vi "agilent_reader.vi"(0 "Action":u8(ring)=1 items=["read new values"=1, "read last values "=2], 5 "Voltage Readings":u16=3, 7 "Temperature Readings":u16=1) -> (1 "Burette Temp Average":dbl, 2 "Cell Temp":dbl, 3 "Acid Temp":dbl, 4 "Burette Temp 1":dbl, 6 "Burette Temp 2":dbl, 8 "Room Temp":dbl, 10 "Voltage 1":dbl, 11 "Data Cluster":T1, 12 "Voltage 1 StandDev":dbl, 13 "Voltage 2 StandDev":dbl, 14 "Average Voltage":dbl, 15 "Voltage 2":dbl)   [LabVIEW 2010]
doc: "This VI is a wrapper for the agilent_action_engine vi's \"read\" action. It makes spitting out the values you need just a bit easier. Just pass in the number of readings for both voltage and temp and do what you will with the resulting data."
uses:
  ProbeClass/TempProbeSet.lvclass
  <vilib>/Analysis/NI_AALBase.lvlib
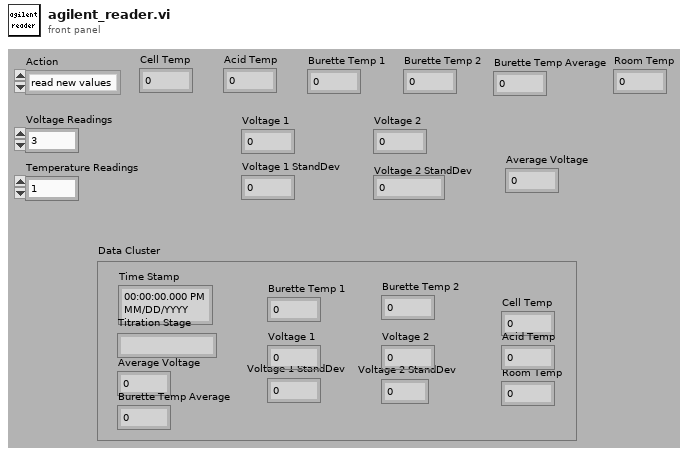
[diagram p1: front panel]
types:
  T1 = cluster{"Time Stamp":timestamp, "Titration Stage":string, "Average Voltage":dbl, "Burette Temp Average":dbl, "Voltage 1":dbl, "Voltage 2":dbl, "Voltage 1 StandDev":dbl, "Voltage 2 StandDev":dbl, "Burette Temp 1":dbl, "Burette Temp 2":dbl, "Cell Temp":dbl, "Acid Temp":dbl, "Room Temp":dbl}
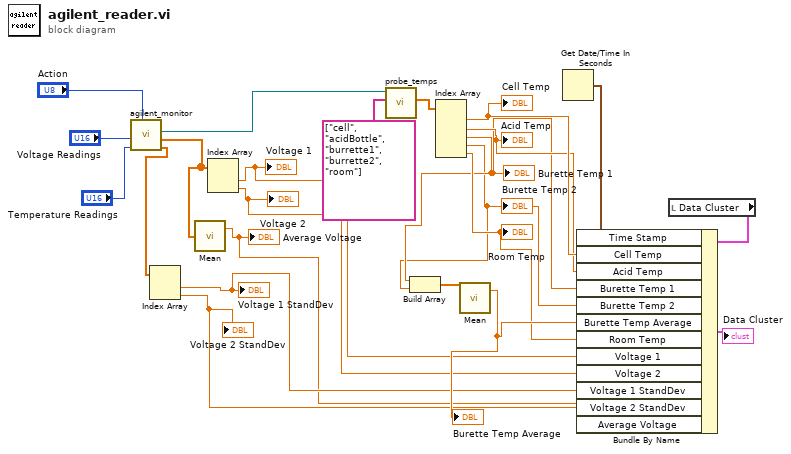
[diagram p0: block diagram]
diagram:
  n1 = call "agilent_monitor.vi"("Action"="Action", "Temperature Readings"="Temperature Readings", "Voltage Readings"="Voltage Readings") -> ("voltage stdvs"=w23:dbl[], "voltages"=w17:dbl[], "TempProbeSet out"=w22:refnum<class "TempProbeSet.lvclass">)  [unwired: 6 in]
  n2 = Index Array(array=w23) -> (element #1=w9:dbl, element #2=w8:dbl)  [unwired: 2 in]
  "Voltage 2 StandDev" <- w8
  "Voltage 1 StandDev" <- w9
  n3 = call <vilib>:"Mean.vi"("X"=w17) -> ("mean"=w7:dbl)  [unwired: 1 out]
  "Average Voltage" <- w7
  n4 = Index Array(array=w17) -> (element #1=w11:dbl, element #2=w10:dbl)  [unwired: 2 in]
  "Voltage 1" <- w11
  "Voltage 2" <- w10
  n5 = call "probe_temps.vi"("locations"=string[] ["cell", "acidBottle", "burrette1", "burrette2", "room"], "TempProbeSet in"=w22) -> ("temps"=w21:dbl[])  [unwired: 7 in, 2 out]
  n6 = Index Array(array=w21) -> (element #1=w4:dbl, element #2=w3:dbl, element #3=w2:dbl, element #4=w1:dbl, element #5=w12:dbl)  [unwired: 5 in]
  "Acid Temp" <- w3
  "Burette Temp 1" <- w2
  "Burette Temp 2" <- w1
  "Cell Temp" <- w4
  "Room Temp" <- w12
  n7 = Build Array(w2, w1) -> (w14:dbl[])
  n8 = call <vilib>:"Mean.vi"("X"=w14) -> ("mean"=w13:dbl)  [unwired: 1 out]
  "Burette Temp Average" <- w13
  n9 = Get Date/Time In Seconds() -> (seconds since 1Jan1904=w5:timestamp)
  n10 = local read "Data Cluster"() -> (w15:T1)
  n11 = Bundle By Name(cluster=w15, "Time Stamp"=w5, "Cell Temp"=w4, "Acid Temp"=w3, "Burette Temp 1"=w2, "Burette Temp 2"=w1, "Burette Temp Average"=w13, "Room Temp"=w12, "Voltage 1"=w11, "Voltage 2"=w10, "Voltage 1 StandDev"=w9, "Voltage 2 StandDev"=w8, "Average Voltage"=w7) -> (→"Data Cluster":T1)
